vi "NXTSumoEyes-DM.vi"(0 "Input of NXTSumoEyes":cluster{"Select Range":u16}={"Select Range"=6} {"Select Range" items=["short"=5, "long"=6]}, 2 "NXT":T4={"error"={"status"=FALSE, "code"=0, "source"=""}, "address"="", "NXT #"=-1, "Show Error"=TRUE, "Connection"=4} {"Connection" items=["USB", "Bluetooth", "USB then Bluetooth", "Last Connection", "Preference"]}, 3 "Input Port":T3 items=["Port 1", "Port 2", "Port 3", "Port 4"]) -> (1 "Output of NXTSumoEyes":T2, 4 "NXT dup":T4={"error"={"status"=FALSE, "code"=0, "source"=""}, "address"="", "NXT #"=-1, "Show Error"=TRUE, "Connection"=4} {"Connection" items=["USB", "Bluetooth", "USB then Bluetooth", "Last Connection", "Preference"]})   [LabVIEW 2009]
uses:
  <vilib>/NXT/Subs/LVHSConnector.ctl
  <vilib>/NXT/Block Support/NXT_InputPort.ctl
  <vilib>/NXT/Block Support/HWPage.SensorMode.ctl
panel:
  in  "Sensor Mode":T1=128 items=["RAWMODE"=0, "BOOLEANMODE"=32, "TRANSITIONCNTMODE"=64, "PERIODCOUNTERMODE"=96, "PCTFULLSCALEMODE"=128, "CELSIUSMODE"=160, "FAHRENHEITMODE"=192, "ANGLESTEPMODE"=224]
  out "Raw Value":i16 caption="Scaled Value"
  in  "Which Zone?":u8
  # "mindsensors.com\nCopyright (c) 2009 by mindsensors.com\nEmail: info (<at>) mindsensors (<dot>) com\n\nThis program is free software. You can redistribute it and/or modify\nit under the terms of the GNU General Public License as published by\nthe Free Software Foundation; version 3 of the License.\nRead the license at: http://www.gnu.org/licenses/gpl.txt"
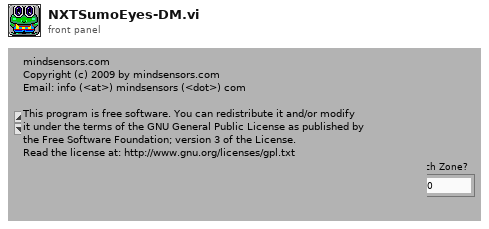
[diagram p1: front panel]
types:
  T1 = typedef "HWPage.SensorMode.ctl" = u8
  T2 = cluster{"Which Zone?":u8, "Scaled Value":i16, "Status":bool}
  T3 = typedef "NXT_InputPort.ctl" = u8
  T4 = typedef "LVHSConnector.ctl" = cluster{"error":errorcluster, "address":string, "NXT #":i32, "Show Error":bool, "Connection":u16}
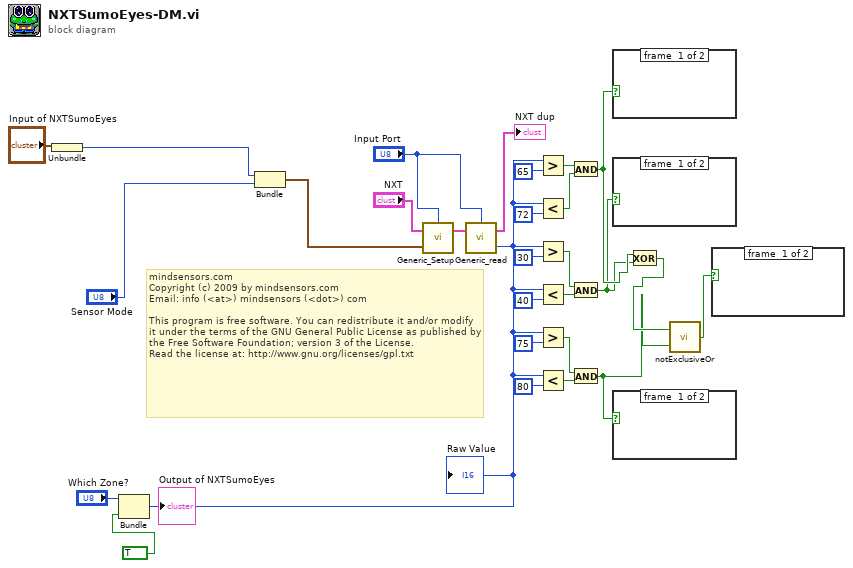
[diagram p0: block diagram]
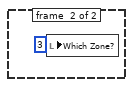
[diagram p2: hidden frame]
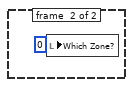
[diagram p3: hidden frame]
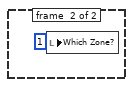
[diagram p4: hidden frame]
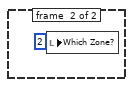
[diagram p5: hidden frame]
diagram:
  # "mindsensors.com\nCopyright (c) 2009 by mindsensors.com\nEmail: info (<at>) mindsensors (<dot>) com\n\nThis program is free software. You can redistribute it and/or modify\nit under the terms of the GNU General Public License as published by\nthe Free Software Foundation; version 3 of the License.\nRead the license at: http://www.gnu.org/licenses/gpl.txt"
  n1 = Unbundle("Input of NXTSumoEyes") -> ("Select Range"=w2:u16)
  n2 = Bundle("Select Range"=w2, "Sensor Mode"="Sensor Mode") -> (w1:cluster{"Select Range":u16, "Sensor Mode":T1})  [unwired: 1 in]
  n3 = call <vilib>:"Generic_Setup.vi"("Sensor Setup"=w1, "NXT"="NXT", "Port"="Input Port") -> ("NXT"=w29:T4)  [unwired: 1 out]
  n4 = call <vilib>:"Generic_read.vi"("NXT"=w29, "Port (Port 3)"="Input Port") -> ("Scaled Value"=w6:i16, "NXT"=→"NXT dup":T4)  [unwired: 1 out]
  "Raw Value" <- w6
  n5 = Bundle("Which Zone?"="Which Zone?", "Scaled Value"=w6, "Status"=TRUE) -> (→"Output of NXTSumoEyes":T2)  [unwired: 1 in]
  n6 = Greater?(x=w6, y=u8 65 ("x")) -> (0:w20:bool)
  n7 = Less?(x=w6, y=u8 72) -> (x < y?=w19:bool)
  n8 = Greater?(x=w6, y=u8 30 ("x")) -> (0:w16:bool)
  n9 = Less?(x=w6, y=u8 40) -> (x < y?=w15:bool)
  n10 = Greater?(x=w6, y=u8 75 ("x")) -> (0:w24:bool)
  n11 = Less?(x=w6, y=u8 80) -> (x < y?=w23:bool)
  n12 = And(x=w20, y=w19) -> (x .and. y?=w12:bool)
  n13 = And(x=w16, y=w15) -> (x .and. y?=w11:bool)
  n14 = And(x=w24, y=w23) -> (x .and. y?=w9:bool)
  n15 = case shown="False" w12 {
    frame #0 {
    }
    frame #1 {
      n16 = local write "Which Zone?"(2) -> ()
    }
  }
  n17 = case shown="False" w11 {
    frame #0 {
    }
    frame #1 {
      n18 = local write "Which Zone?"(1) -> ()
    }
  }
  n19 = case shown="False" w9 {
    frame #0 {
    }
    frame #1 {
      n20 = local write "Which Zone?"(0) -> ()
    }
  }
  n21 = Exclusive Or(1:w11, 2:w12) -> (0:w10:bool)
  n22 = call <vilib>:"notExclusiveOr.vi"("y"=w9, "x"=w10) -> (".not. (x xor. y)?"=w8:bool)
  n23 = case shown="True" w8 {
    frame #0 {
    }
    frame #1 {
      n24 = local write "Which Zone?"(3) -> ()
    }
  }
